vi "single sweep - setup fast F sweep.vi"(4 "TO, ms":u32=100, 5 "Retry on TO":bool, 8 "error in":errorcluster, 11 "RUS settings in":T1={"NI-DAQ lockin settings"={"Samples per sine wave"=0, "Sine waves per freq step"=0, "Output Representation"=enum."Real/Imaginary", "Low-pass filter"=enum."Butterworth", "Ranges and couplings "=[]}, "Fast swep settings"={"Update rate (Hz)"=250.0, "Start F, Hz"=200000.0, "Stop F"=1700000.0, "Number of points"=30000, "Amplitude"=2.1, "Init&amplitude"=TRUE, "IF"=1000.0, "Time constant"=0.1}, "Pre-sweep delay, s"=0.0, "Lockin mode"=enum."NI-DAQ", "SR Lockin"="GPIB0::10::INSTR", "DAQmx Device"="Dev3", "Clock Multiplier"=64, "Fast Sweep Data Out"={"DO clock task"="", "DO task"="", "Update clock task"="", "DAQ lockin task"="", "Pre-sweep counter task"=""}, "Lockin Range, V"=0.0, "F Array"=[], "Freq. update clock terminal"="", "DO Clock Rate (Hz)"=5000000.0, "ADC clock terminal"="/PFI4", "Pre-sweep counter terminal"="/PFI4", "Samples per read"=10, "DO clock terminal"="", "Pre-sweep points"=0, "F points per write"=0, "Total sweep time, s"=1000.0, "Initial SYNTH phase"=0.0, "Record IF"=FALSE, "Save data settings"={"Save data"=TRUE, "Data Root Path"=path "", "File Prefix"="", "File Format"=enum."ASCII", "Save column names"=TRUE, "File Comments"="<Description of the current file>", "User/Prj"="<User Name/Project Description>"}, "Data file path"=path "", "New data user event"=refnum, "Stop user event"=refnum, "Number of channels"=1, "Auto-phase"=FALSE} {"Lockin Range, V" format="%#_6e"; "Fast swep settings"."IF" format="%#_6p"; "Fast swep settings"."Amplitude" min=0.0 max=2.5; "Fast swep settings"."Number of points" format="%.0p"; "Fast swep settings"."Stop F" format="%#_6p"; "Fast swep settings"."Start F, Hz" format="%#_6p"; "Fast swep settings"."Update rate (Hz)" format="%0.2f"; "NI-DAQ lockin settings"."Ranges and couplings"."Coupling" items=["default"=-1, "RSE"=10083, "NRSE"=10078, "Differential"=10106, "Pseudodifferential"=12529]}) -> (0 "error out":errorcluster, 3 "RUS settings out":T1={"NI-DAQ lockin settings"={"Samples per sine wave"=0, "Sine waves per freq step"=0, "Output Representation"=enum."Real/Imaginary", "Low-pass filter"=enum."Butterworth", "Ranges and couplings "=[]}, "Fast swep settings"={"Update rate (Hz)"=250.0, "Start F, Hz"=200000.0, "Stop F"=1700000.0, "Number of points"=30000, "Amplitude"=2.1, "Init&amplitude"=TRUE, "IF"=1000.0, "Time constant"=0.1}, "Pre-sweep delay, s"=0.0, "Lockin mode"=enum."NI-DAQ", "SR Lockin"="GPIB0::10::INSTR", "DAQmx Device"="Dev3", "Clock Multiplier"=64, "Fast Sweep Data Out"={"DO clock task"="", "DO task"="", "Update clock task"="", "DAQ lockin task"="", "Pre-sweep counter task"=""}, "Lockin Range, V"=0.0, "F Array"=[], "Freq. update clock terminal"="", "DO Clock Rate (Hz)"=5000000.0, "ADC clock terminal"="/PFI4", "Pre-sweep counter terminal"="/PFI4", "Samples per read"=10, "DO clock terminal"="", "Pre-sweep points"=0, "F points per write"=0, "Total sweep time, s"=1000.0, "Initial SYNTH phase"=0.0, "Record IF"=FALSE, "Save data settings"={"Save data"=TRUE, "Data Root Path"=path "", "File Prefix"="", "File Format"=enum."ASCII", "Save column names"=TRUE, "File Comments"="<Description of the current file>", "User/Prj"="<User Name/Project Description>"}, "Data file path"=path "", "New data user event"=refnum, "Stop user event"=refnum, "Number of channels"=1, "Auto-phase"=FALSE} {"Lockin Range, V" format="%#_6e"; "Fast swep settings"."IF" format="%#_6p"; "Fast swep settings"."Amplitude" min=0.0 max=2.5; "Fast swep settings"."Number of points" format="%.0p"; "Fast swep settings"."Stop F" format="%#_6p"; "Fast swep settings"."Start F, Hz" format="%#_6p"; "Fast swep settings"."Update rate (Hz)" format="%0.2f"; "NI-DAQ lockin settings"."Ranges and couplings"."Coupling" items=["default"=-1, "RSE"=10083, "NRSE"=10078, "Differential"=10106, "Pseudodifferential"=12529]})   [LabVIEW 2010]
uses:
  RUS/Controls/RUS settings.ctl
  RUS/Controls/RUS NI-DAQ Lockin Settings.ctl
  RUS/Controls/Sweep settings.ctl
  File/Controls/Save data settings.ctl
  File/Controls/File formats.ctl
panel:
  out "DO task setup time":u32
  out "F1 out time":u32
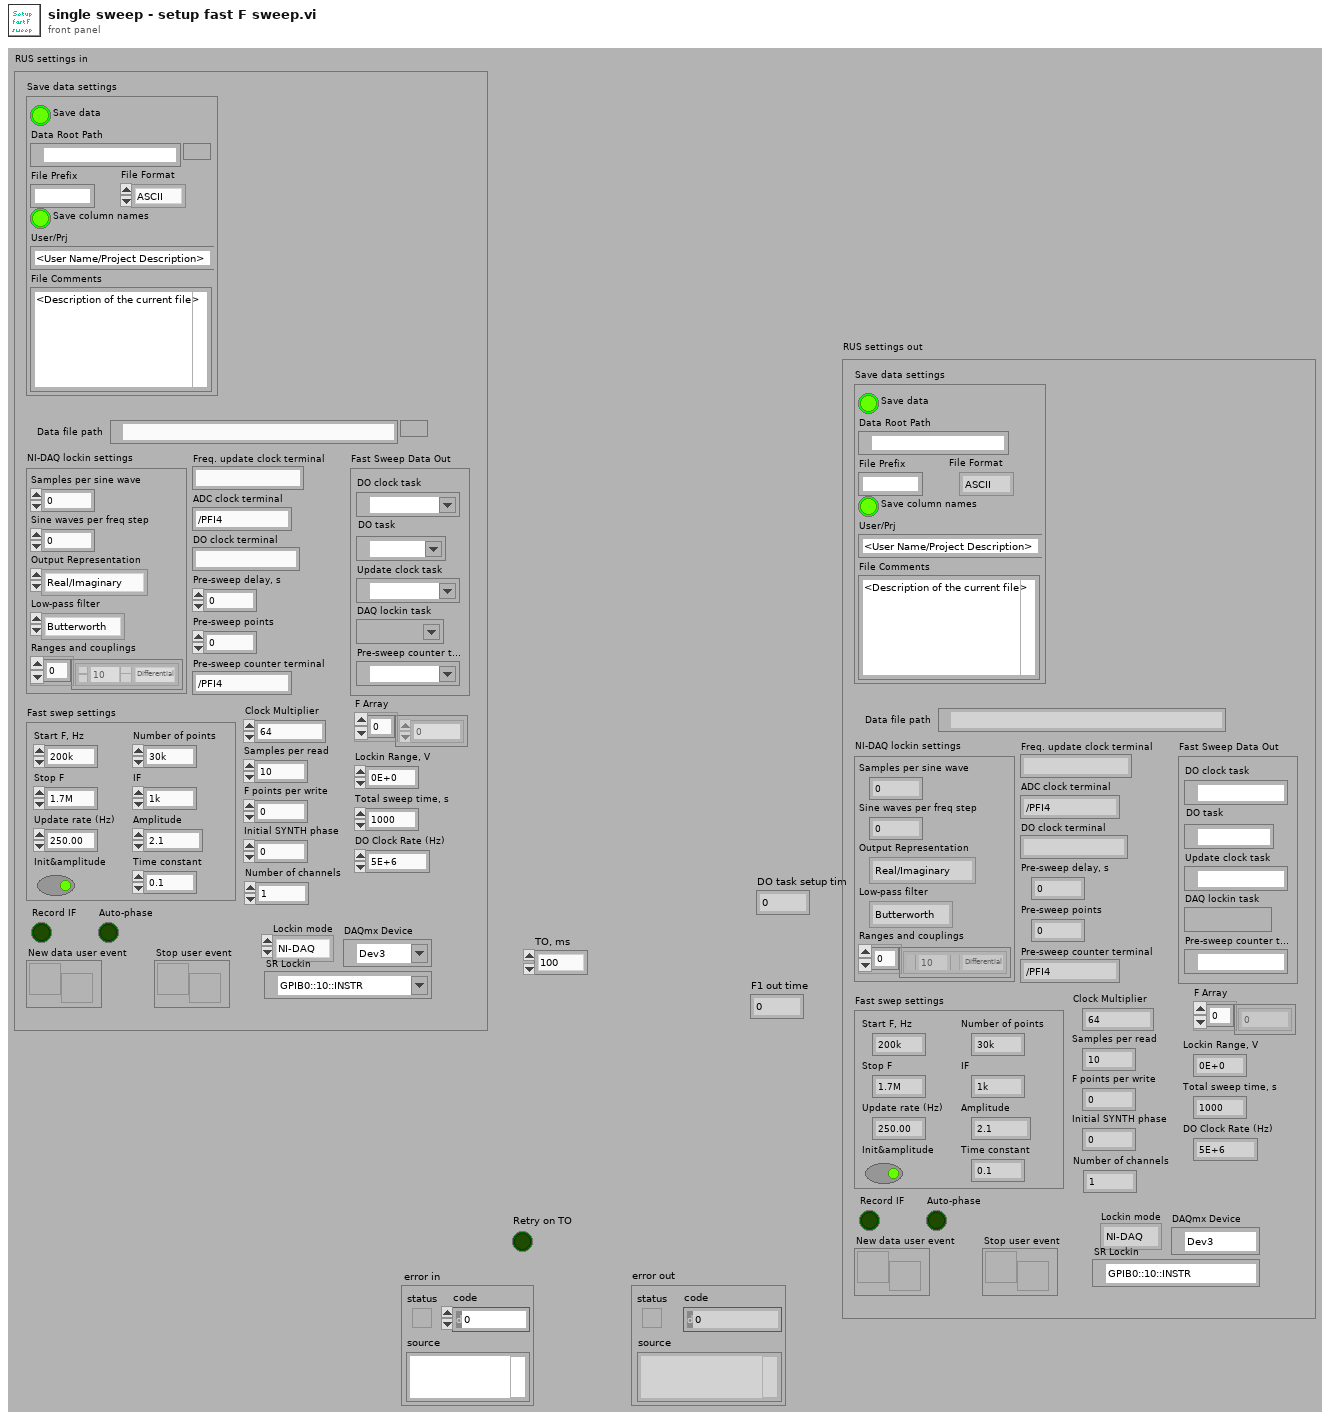
[diagram p1: front panel]
types:
  T1 = typedef "RUS settings.ctl" = cluster{"NI-DAQ lockin settings":T2, "Fast swep settings":T3, "Pre-sweep delay, s":dbl, "Lockin mode":enum16{"SRS", "NI-DAQ"}, "SR Lockin":refnum<visa-resource-name>, "DAQmx Device":tag, "Clock Multiplier":i32, "Fast Sweep Data Out":cluster{"DO clock task":refnum<k21>, "DO task":refnum<k21>, "Update clock task":refnum<k21>, "DAQ lockin task":refnum<k21>, "Pre-sweep counter task":refnum<k21>}, "Lockin Range, V":sgl, "F Array":dbl[], "Freq. update clock terminal":string, "DO Clock Rate (Hz)":dbl, "ADC clock terminal":string, "Pre-sweep counter terminal":string, "Samples per read":i32, "DO clock terminal":string, "Pre-sweep points":i32, "F points per write":i32, "Total sweep time, s":dbl, "Initial SYNTH phase":dbl, "Record IF":bool, "Save data settings":T4, "Data file path":path, "New data user event":refnum<user-event>, "Stop user event":refnum<user-event>, "Number of channels":i32, "Auto-phase":bool}
  T2 = typedef "RUS NI-DAQ Lockin Settings.ctl" = cluster{"Samples per sine wave":i32, "Sine waves per freq step":i32, "Output Representation":enum16{"Real/Imaginary", "Polar"}, "Low-pass filter":enum16{"No filtering", "Butterworth", "Bessel"}, "Ranges and couplings ":cluster{"Range":dbl, "Coupling":i32}[]}
  T3 = typedef "Sweep settings.ctl" = cluster{"Update rate (Hz)":dbl, "Start F, Hz":dbl, "Stop F":dbl, "Number of points":i32, "Amplitude":dbl, "Init&amplitude":bool, "IF":dbl, "Time constant":dbl}
  T4 = typedef "Save data settings.ctl" = cluster{"Save data":bool, "Data Root Path":path, "File Prefix":string, "File Format":T5, "Save column names":bool, "File Comments":string, "User/Prj":string}
  T5 = typedef "File formats.ctl" = enum16{"TDMS", "ASCII", "BINARY"}
  T6 = enum16{"Direct, clock*f1", "Direct, clock*f2", "Heterodyne"}
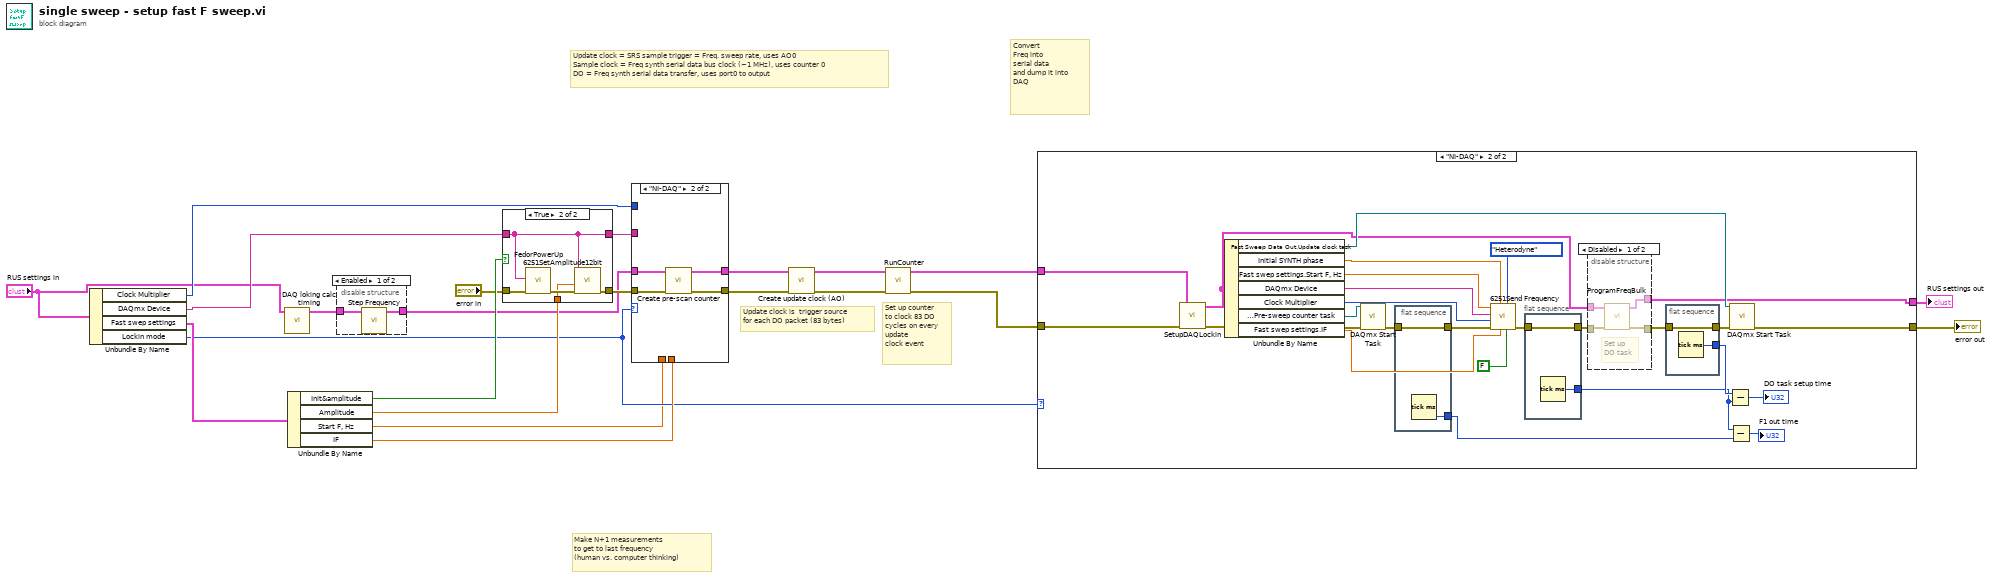
[diagram p0: block diagram]
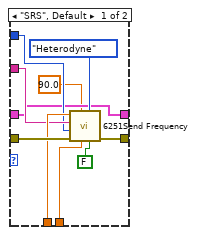
[diagram p3: hidden frame]
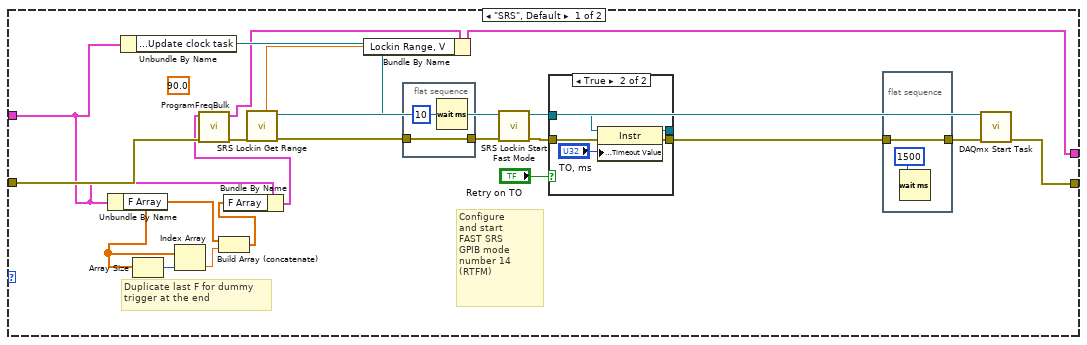
[diagram p4: hidden frame]
diagram:
  # "Make N+1 measurements\nto get to last frequency\n(human vs. computer thinking)"
  # "Set up counter\nto clock 83 DO\ncycles on every\nupdate \nclock event"
  # "Convert \nFreq into \nserial data \nand dump it into \nDAQ"
  # "Update clock is  trigger source\nfor each DO packet (83 bytes)"
  # "Update clock = SRS sample trigger = Freq. sweep rate, uses AO0\nSample clock = Freq synth serial data bus clock (~1 MHz), uses counter 0\nDO = Freq synth serial data transfer, uses port0 to output"
  n1 = Unbundle By Name("RUS settings in") -> ("Clock Multiplier"=w8:i32, "DAQmx Device"=w11:tag, "Fast swep settings"=w13:T3, "Lockin mode"=w12:enum16{"SRS", "NI-DAQ"})
  n2 = call "DAQ loking calc timing.vi"("RUS settings"="RUS settings in") -> ("RUS settings out"=w4:T1)  [unwired: 10 in]
  n3 = Unbundle By Name(w13) -> ("Init&amplitude"=w21:bool, "Amplitude"=w22:dbl, "Start F, Hz"=w6:dbl, "IF"=w16:dbl)
  n4 = disable-structure shown="Enabled" {
    disable-tunnel: w4 -> [w24 w25]
    disable-tunnel: [w23 w25] -> w2
    frame Enabled {
      n5 = call "Step Frequency.vi"("RUS settings"=w24) -> ("RUS settings out"=w23:T1)  [unwired: 3 in, 7 out]
    }
    frame Disabled {
    }
  }
  n6 = case shown="True" w21 {
    tunnel: "error in" -> [w27 w32]
    tunnel: [w27 w30] -> w19
    tunnel: w11 -> [w26 w29]
    tunnel: [w26 w29] -> w17
    tunnel: w22 -> [_ w28]
    frame False {
    }
    frame True {
      n7 = call "FedorPowerUp.vi"("error in (no error)"=w32, "DAQmx Device Name"=w29) -> ("error out"=w31:errorcluster)  [unwired: 9 out]
      n8 = call "6251SetAmplitude12bit.vi"("error in (no error)"=w31, "0 to 2.1 VRMS"=w28, "DAQmx Device Name"=w29) -> ("error out"=w30:errorcluster)  [unwired: 8 out]
    }
  }
  n9 = case shown="\"NI-DAQ\"" w12 {
    tunnel: w19 -> [w42 w46]
    tunnel: [w41 w45] -> w3
    tunnel: w16 -> [w40 _]
    tunnel: w6 -> [w38 _]
    tunnel: w17 -> [w37 _]
    tunnel: w8 -> [w36 _]
    tunnel: w2 -> [w34 w44]
    tunnel: [w34 w43] -> w1
    frame "SRS", Default {
      n10 = call "6251Send Frequency.vi"("Use hardware clock for DO"=FALSE ("6251"), "Mode"=T6."Heterodyne", "IF (Hz)"=w40, "Phase (degrees)"=90.0, "error in (no error)"=w42, "Clock Multiplier"=w36, "DAQmx Device Name"=w37, "f (Hz)"=w38) -> ("error out"=w41:errorcluster)  [unwired: 3 out]
    }
    frame "NI-DAQ" {
      n11 = call "Create pre-scan counter.vi"("error in"=w46, "RUS settings"=w44) -> ("error out"=w45:errorcluster, "RUS settings out"=w43:T1)  [unwired: 8 in]
    }
  }
  n12 = call "Create update clock (AO).vi"("error in"=w3, "RUS settings"=w1) -> ("error out"=w18:errorcluster, "RUS settings out"=w10:T1)  [unwired: 3 in, 5 out]
  n13 = call "RunCounter.vi"("error in (no error)"=w18, "RUS settings"=w10) -> ("error out"=w15:errorcluster, "RUS settings out"=w9:T1)  [unwired: 2 in, 6 out]
  n14 = case shown="\"NI-DAQ\"" w12 {
    tunnel: w15 -> [w54 w104]
    tunnel: [w58 w90] -> w14
    tunnel: w9 -> [w49 w79]
    tunnel: [w56 w85] -> w5
    frame "SRS", Default {
      (unwired) 90.0 ("Phase (degrees)")
      # "Duplicate last F for dummy \ntrigger at the end"
      # "Configure \nand start \nFAST SRS\nGPIB mode\nnumber 14\n(RTFM)"
      n15 = Unbundle By Name(w49) -> ("F Array"=w50:dbl[])
      n16 = Unbundle By Name(w49) -> ("Fast Sweep Data Out.Update clock task"=w57:refnum<k21>)
      n17 = Array Size(array=w50) -> (size(s)=w51:i32)
      n18 = Index Array(array=w50, index=w51) -> (element=w52:dbl)
      n19 = Build Array (concatenate)(w50, w52) -> (w48:dbl[])
      n20 = Bundle By Name(cluster=w49, "F Array"=w48) -> (w47:T1)
      n21 = call "ProgramFreqBulk.vi"("error in (no error)"=w54, "RUS settings"=w47) -> ("error out"=w61:errorcluster, "RUS settings out"=w53:T1)  [unwired: 3 in, 5 out]
      n22 = call "SRS Lockin Get Range.vi"("error in (no error)"=w61) -> ("error out"=w63:errorcluster, "VISA resource name out"=w67:refnum<visa-resource-name>, "Range, V"=w55:sgl)  [unwired: 1 in, 7 out]
      n23 = Bundle By Name(cluster=w53, "Lockin Range, V"=w55) -> (w56:T1)
      n24 = flat-sequence {
        tunnel: w63 -> [w71]
        tunnel: [w71] -> w62
        frame #0 {
          n25 = Wait (ms)(milliseconds to wait=u32 10) -> ()  [unwired: 1 out]
        }
      }
      n26 = call "SRS Lockin Start Fast Mode.vi"("error in (no error)"=w62, "VISA Resource Name"=w67) -> ("error out"=w66:errorcluster, "VISA resource name out"=w64:refnum<visa-resource-name>)  [unwired: 1 in, 7 out]
      n27 = case shown="True" "Retry on TO" {
        tunnel: w66 -> [w73 w78]
        tunnel: [w73 w77] -> w60
        tunnel: w64 -> [w72 w75]
        tunnel: [w72 w74] -> _
        frame False {
        }
        frame True {
          n28 = property class="Instr"(reference=w75, error in=w78, "General Settings:Timeout Value"="TO, ms") -> (reference out=w74:refnum<visa-resource-name>, error out=w77:errorcluster)
        }
      }
      n29 = flat-sequence {
        tunnel: w60 -> [w69]
        tunnel: [w69] -> w59
        frame #0 {
          n30 = Wait (ms)(milliseconds to wait=u32 1500) -> ()  [unwired: 1 out]
        }
      }
      n31 = call <vilib>:"DAQmx Start Task.vi"("task/channels in"=w57, "error in"=w59) -> ("error out"=w58:errorcluster)  [unwired: 13 out]
    }
    frame "NI-DAQ" {
      n32 = call "SetupDAQLockin.vi"("error in (no error)"=w104, "RUS settings"=w79) -> ("error out"=w91:errorcluster, "RUS settings out"=w86:T1)  [unwired: 8 in]
      n33 = Unbundle By Name(w86) -> ("Fast Sweep Data Out.Update clock task"=w89:refnum<k21>, "Initial SYNTH phase"=w80:dbl, "Fast swep settings.Start F, Hz"=w83:dbl, "DAQmx Device"=w88:tag, "Clock Multiplier"=w82:i32, "Fast Sweep Data Out.Pre-sweep counter task"=w92:refnum<k21>, "Fast swep settings.IF"=w84:dbl)
      n34 = call <vilib>:"DAQmx Start Task.vi"("task/channels in"=w92, "error in"=w91) -> ("error out"=w97:errorcluster)  [unwired: 13 out]
      n35 = flat-sequence {
        tunnel: w97 -> [w112]
        tunnel: [w112] -> w96
        tunnel: [w111] -> w94
        frame #0 {
          n36 = Tick Count (ms)() -> (millisecond timer value=w111:u32)
        }
      }
      n37 = call "6251Send Frequency.vi"("Use hardware clock for DO"=FALSE ("6251"), "Mode"=T6."Heterodyne", "IF (Hz)"=w84, "Phase (degrees)"=w80, "error in (no error)"=w96, "Clock Multiplier"=w82, "DAQmx Device Name"=w88, "f (Hz)"=w83) -> ("error out"=w101:errorcluster)  [unwired: 3 out]
      n38 = flat-sequence {
        tunnel: w101 -> [w116]
        tunnel: [w116] -> w87
        tunnel: [w115] -> w81
        frame #0 {
          n39 = Tick Count (ms)() -> (millisecond timer value=w115:u32)
        }
      }
      n40 = disable-structure shown="Disabled" {
        disable-tunnel: [w108 w109] -> w100
        disable-tunnel: w87 -> [w107 w109]
        disable-tunnel: w86 -> [w106 w110]
        disable-tunnel: [w105 w110] -> w85
        frame Disabled {
          # "Set up\nDO task"
          n41 = call "ProgramFreqBulk.vi"("error in (no error)"=w107, "RUS settings"=w106) -> ("error out"=w108:errorcluster, "RUS settings out"=w105:T1)  [unwired: 3 in, 5 out]
        }
        frame Enabled {
        }
      }
      n42 = flat-sequence {
        tunnel: w100 -> [w114]
        tunnel: [w114] -> w99
        tunnel: [w113] -> w95
        frame #0 {
          n43 = Tick Count (ms)() -> (millisecond timer value=w113:u32)
        }
      }
      n44 = Subtract(x=w95, y=w81) -> (x-y=→"DO task setup time":u32)
      n45 = Subtract(x=w81, y=w94) -> (x-y=→"F1 out time":u32)
      n46 = call <vilib>:"DAQmx Start Task.vi"("task/channels in"=w89, "error in"=w99) -> ("error out"=w90:errorcluster)  [unwired: 12 in, 1 out]
    }
  }
  "error out" <- w14
  "RUS settings out" <- w5
